vi "GetClassCluster.vi"(8 "error in (no error)":errorcluster, 10 "Experiment Data":T1, 11 "Experiment.lvclass":refnum<class "Experiment.lvclass">) -> (0 "error out":errorcluster, 3 "Experiment.lvclass Out":refnum<class "Experiment.lvclass">)   [LabVIEW 2019, in "Experiment.lvclass"]
uses:
  Experiment.lvclass
  ClassCluster.ctl
  DevicesClass/BaseDevice/BaseDevice.lvclass
  Experiment.lvclass/Experiment.ctl
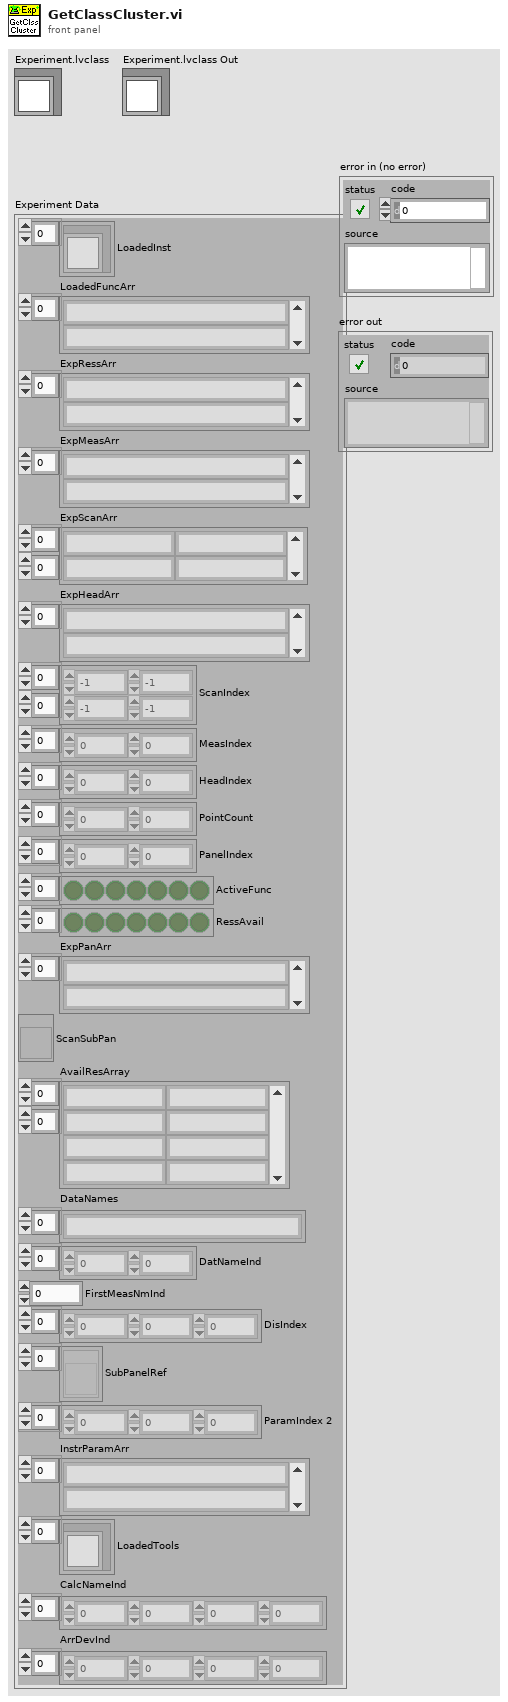
[diagram p1: front panel]
types:
  T1 = typedef "ClassCluster.ctl" = cluster{"LoadedInst":refnum<class "BaseDevice.lvclass">[], "LoadedFuncArr":string[], "ExpRessArr":string[], "ExpMeasArr":string[], "ExpScanArr":string[][], "ExpHeadArr":string[], "ScanIndex":i32[][], "MeasIndex":i32[], "HeadIndex":i32[], "PointCount":i32[], "PanelIndex":i32[], "ActiveFunc":bool[], "RessAvail":bool[], "ExpPanArr":string[], "ScanSubPan":refnum<vi>, "AvailResArray":string[][], "DataNames":string[], "DatNameInd":i32[], "FirstMeasNmInd":i32, "DisIndex":i32[], "SubPanelRef":refnum<vi>[], "ParamIndex 2":i32[], "InstrParamArr":string[], "LoadedTools":refnum<class "BaseDevice.lvclass">[], "CalcNameInd":i32[], "ArrDevInd":i32[]}
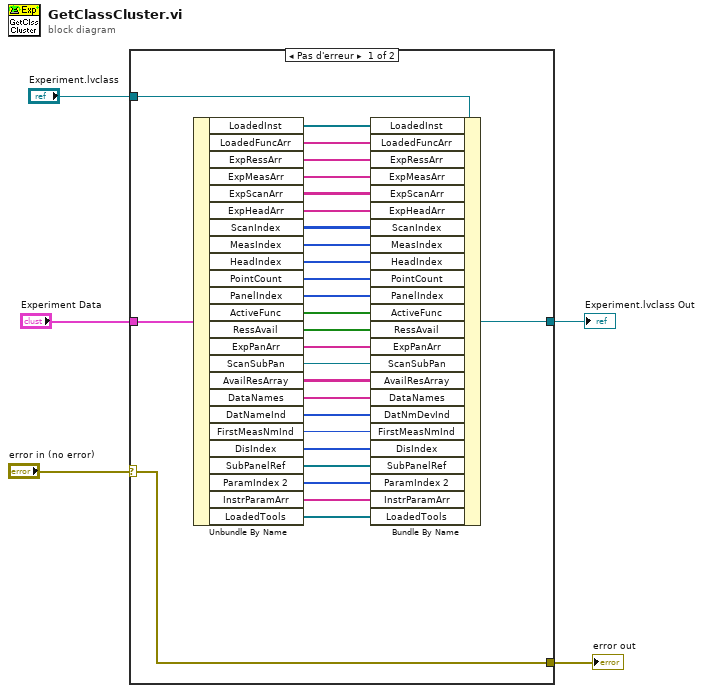
[diagram p0: block diagram]
diagram:
  n1 = case shown="Pas d'erreur" "error in (no error)" {
    selector: "error in (no error)" -> [w9 w34]
    tunnel: "Experiment.lvclass" -> [w7 w35]
    tunnel: [w9 w34] -> w3
    tunnel: [w6 w35] -> w2
    tunnel: "Experiment Data" -> [w8 _]
    frame No Error {
      n2 = Unbundle By Name(w8) -> ("LoadedInst"=w33:refnum<class "BaseDevice.lvclass">[], "LoadedFuncArr"=w32:string[], "ExpRessArr"=w31:string[], "ExpMeasArr"=w30:string[], "ExpScanArr"=w29:string[][], "ExpHeadArr"=w28:string[], "ScanIndex"=w27:i32[][], "MeasIndex"=w26:i32[], "HeadIndex"=w25:i32[], "PointCount"=w24:i32[], "PanelIndex"=w23:i32[], "ActiveFunc"=w22:bool[], "RessAvail"=w21:bool[], "ExpPanArr"=w20:string[], "ScanSubPan"=w19:refnum<vi>, "AvailResArray"=w18:string[][], "DataNames"=w17:string[], "DatNameInd"=w16:i32[], "FirstMeasNmInd"=w15:i32, "DisIndex"=w14:i32[], "SubPanelRef"=w13:refnum<vi>[], "ParamIndex 2"=w12:i32[], "InstrParamArr"=w11:string[], "LoadedTools"=w10:refnum<class "BaseDevice.lvclass">[])
      n3 = Bundle By Name(cluster=w7, "LoadedInst"=w33, "LoadedFuncArr"=w32, "ExpRessArr"=w31, "ExpMeasArr"=w30, "ExpScanArr"=w29, "ExpHeadArr"=w28, "ScanIndex"=w27, "MeasIndex"=w26, "HeadIndex"=w25, "PointCount"=w24, "PanelIndex"=w23, "ActiveFunc"=w22, "RessAvail"=w21, "ExpPanArr"=w20, "ScanSubPan"=w19, "AvailResArray"=w18, "DataNames"=w17, "DatNmDevInd"=w16, "FirstMeasNmInd"=w15, "DisIndex"=w14, "SubPanelRef"=w13, "ParamIndex 2"=w12, "InstrParamArr"=w11, "LoadedTools"=w10) -> (w6:refnum<class "Experiment.lvclass">)
    }
    frame Error {
    }
  }
  "Experiment.lvclass Out" <- w2
  "error out" <- w3
